vi "PwrCal.vi"(7 "VISA":string, 8 "error in (no error)":errorcluster, 9 "RL":dbl, 10 "Port":i32, 11 "type":i32) -> (0 "error out":errorcluster, 3 "return type":i32)   [LabVIEW 2015, in "QCA_DUT_Func.lvlib"]
uses:
  QCA_DUT_Func.lvlib
  QCA_DUT_Func.dll
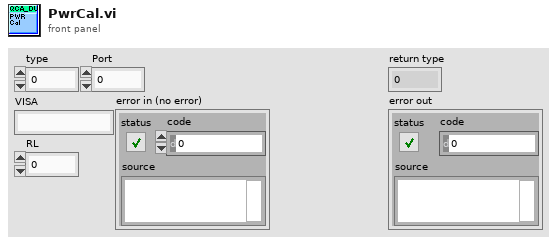
[diagram p1: front panel]
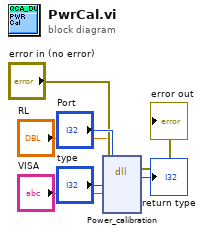
[diagram p0: block diagram]
diagram:
  n1 = dll-call lib="D:/4-Up-WLAN-Test-System/DUT Control/DUT/dut_control/QCA_DUT_Func.dll" fn="Power_calibration"(error in="error in (no error)", "type"="type", "VISA"="VISA", "Port"="Port", "RL"="RL") -> (error out=→"error out":errorcluster, "return type"=→"return type":i32)  [unwired: 6 in, 1 out]
